vi "AXI-Stream-Tester-Top.vi"() -> ()   [LabVIEW 2017]
uses:
  AXI-Stream.States.ctl
  <vilib>/FPGAPlugInAG/PXIe-6592R/niLvFpga_Open_PXIe-6592R.vi
  <vilib>/rvi/interface/common/dynamic/niFpgaDynamicAddResources.vi
  AXI-Stream.Globals.vi
  <vilib>/Utility/error.llb/Error Cluster From Error Code.vi
  <vilib>/rvi/errors/niLvFpgaAdjustHostInterfaceError.vi
  <vilib>/FPGAPlugInAG/Dynamic/niLvFpga_Close_Dynamic.vi
  <vilib>/rvi/interface/nirviOpenFPGA/nirviOpenFPGA.xnode
  FPGA Bitfiles/03MicroBlazeAXIS_FPGATarget_Fpga-AXI-Stream_rt9YWQdBu5Q.lvbitx
  <vilib>/rvi/interface/nirviReadWriteControl/nirviReadWriteControl.xnode
  <vilib>/rvi/interface/nirviMethod/nirviMethod.xnode
  <vilib>/rvi/interface/nirviCloseFPGA/nirviCloseFPGA.xnode
  <vilib>/rvi/errors/niLvFpgaMergeErrorWithErrorCode.vi
  <vilib>/FPGAPlugInAG/Dynamic/niLvFpga_ReadFifo_Dynamic.vi
  <vilib>/rvi/interface/Simulation/niFpgaSimulationCallBeginRW.vi
  <vilib>/FPGAPlugInAG/Dynamic/niLvFpga_WriteFifo_Dynamic.vi
  NiFpgaLv.dll
panel:
  out "AXI_STR_RXD_tready_Count":u16
  out "TXD_tkeep_count 2":u32
  in  "AXI_STR_RXD_tuser":fxp<+,4,4>
  in  "AXI_STR_RXD_tkeep":fxp<+,4,4>
  out "AXI_STR_TXD_tuser":fxp<+,4,4>
  out "AXI_STR_TXD_tkeep":fxp<+,4,4>
  out "TXD_tkeep_count":u32
  out "TXD_tuser_count":u32
  in  "Clear?":bool
  out "GPIO #1 out":u32 format="%.0x"
  in  "GPIO #1 in":u32 format="%.0x"
  in  "Read from GPIO":bool
  in  "Write to GPIO":bool
  in  "Read from FIFO":bool
  out "error out":errorcluster
  out "Read Data":u32[](array[numeric]) format="%.0x"
  in  "DataToSend":u32[](array[numeric])=[240, 241, 242, 243, 244, 245] format="%.0x"
  in  "Send to FIFO":bool
  in  "Stop":bool
  in  "error in":errorcluster
  # "Send a packet of data, read the same data\necho'd back by MicroBlaze MCS"
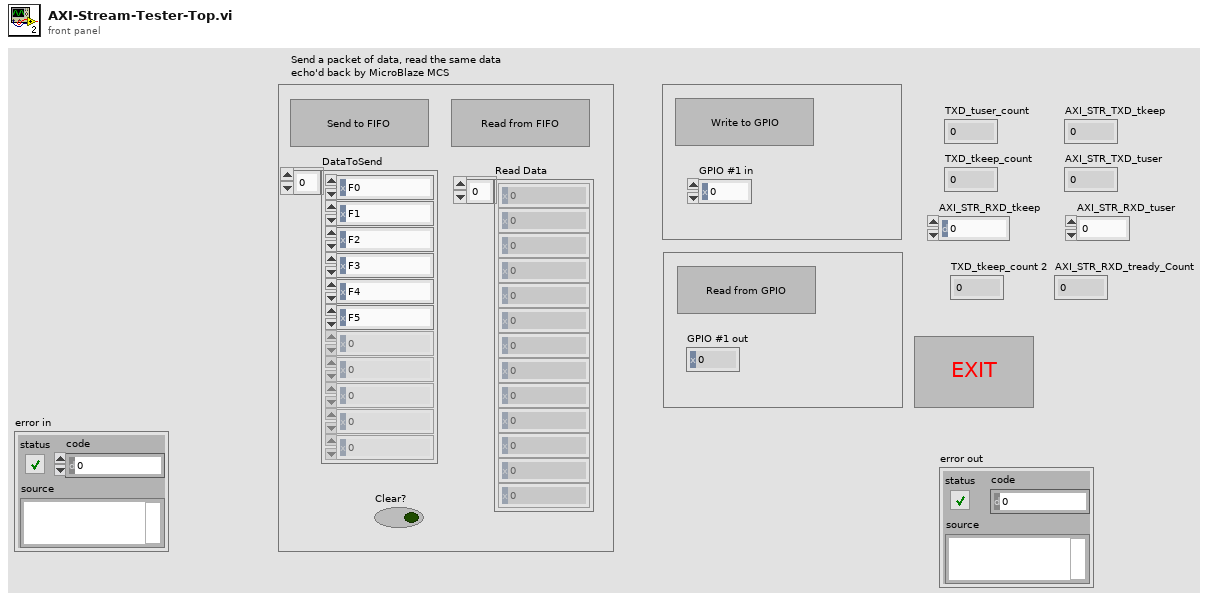
[diagram p1: front panel]
types:
  T1 = typedef "AXI-Stream.States.ctl" = enum16{"Open FPGA", "Send to FIFO", "Read from FIFO", "Write to GPIO", "Read GPIO", "Close FPGA"}
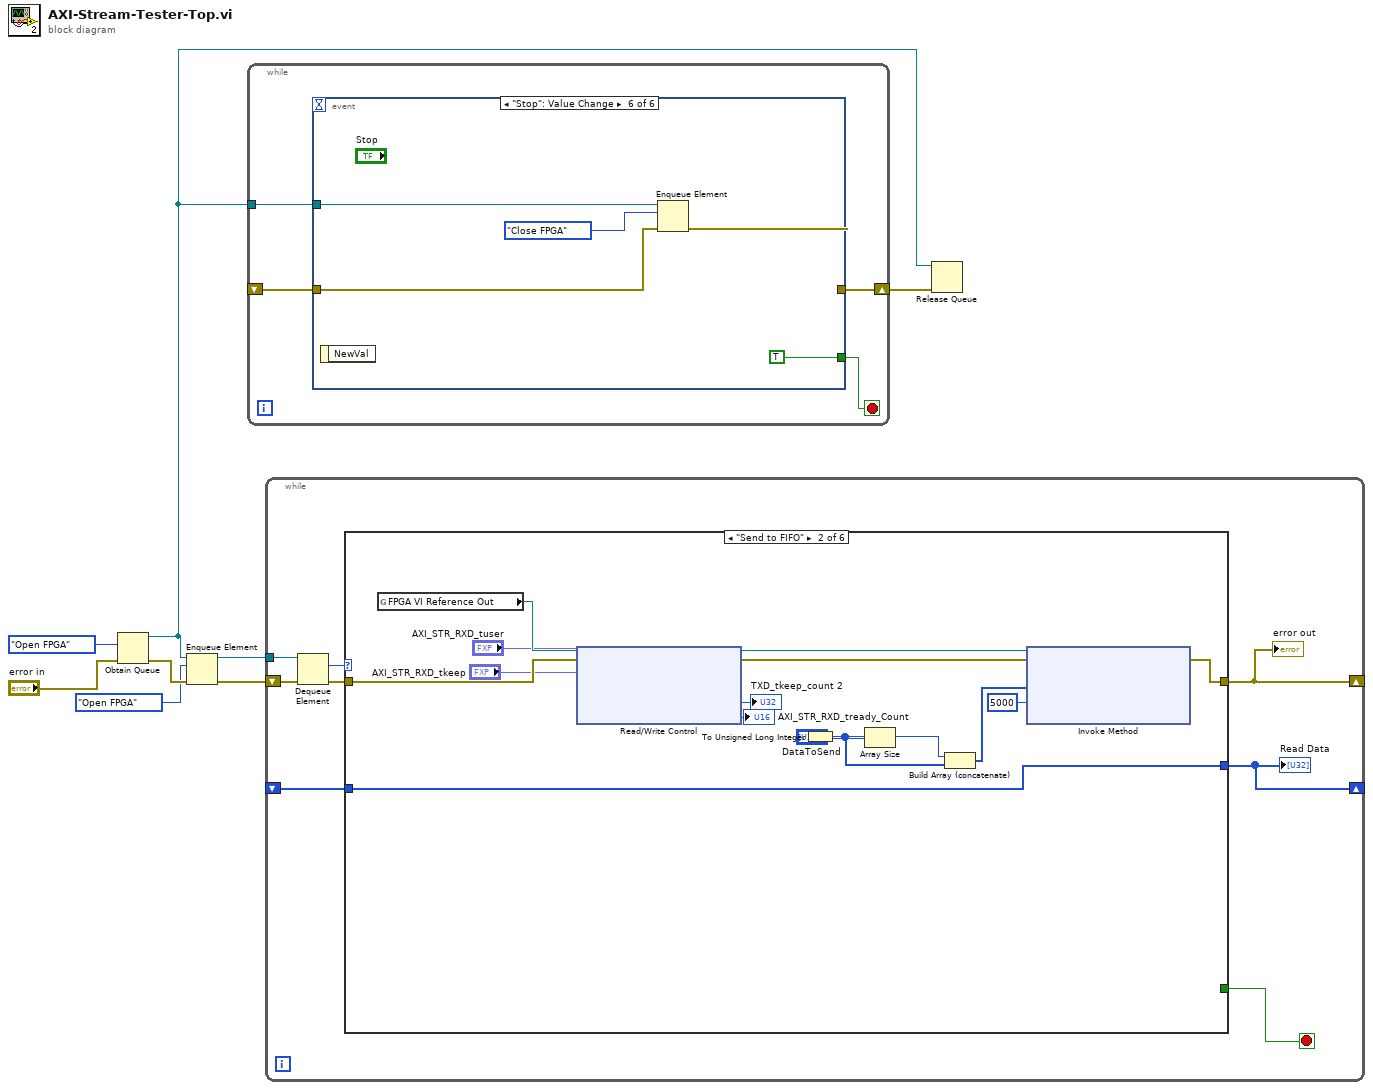
[diagram p0: block diagram]
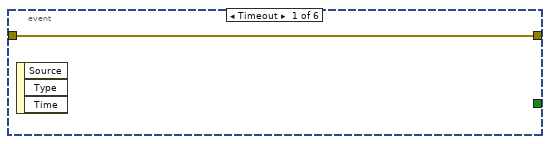
[diagram p2: hidden frame]
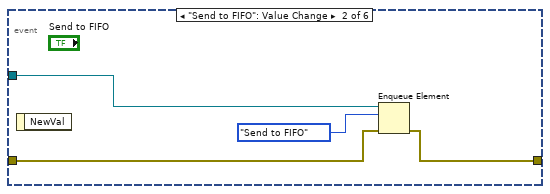
[diagram p3: hidden frame]
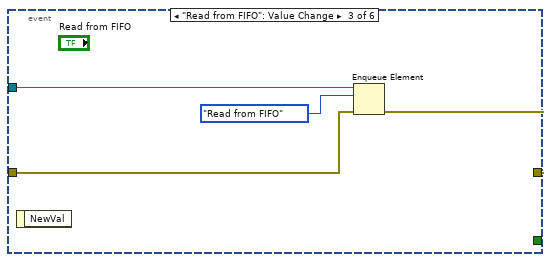
[diagram p4: hidden frame]
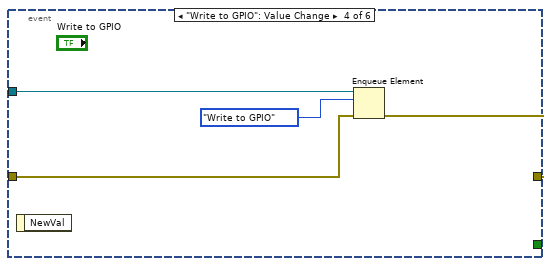
[diagram p5: hidden frame]
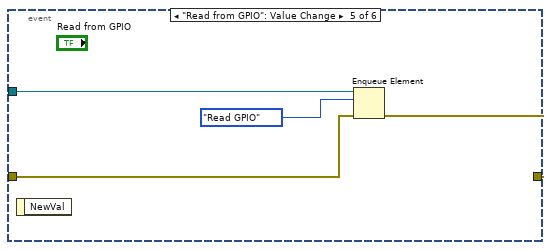
[diagram p6: hidden frame]
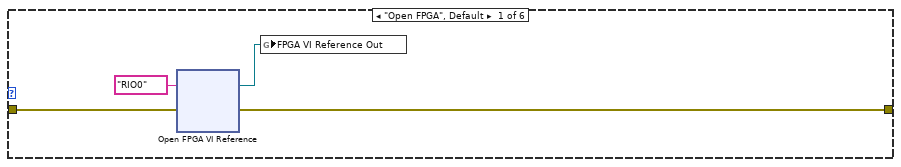
[diagram p7: hidden frame]
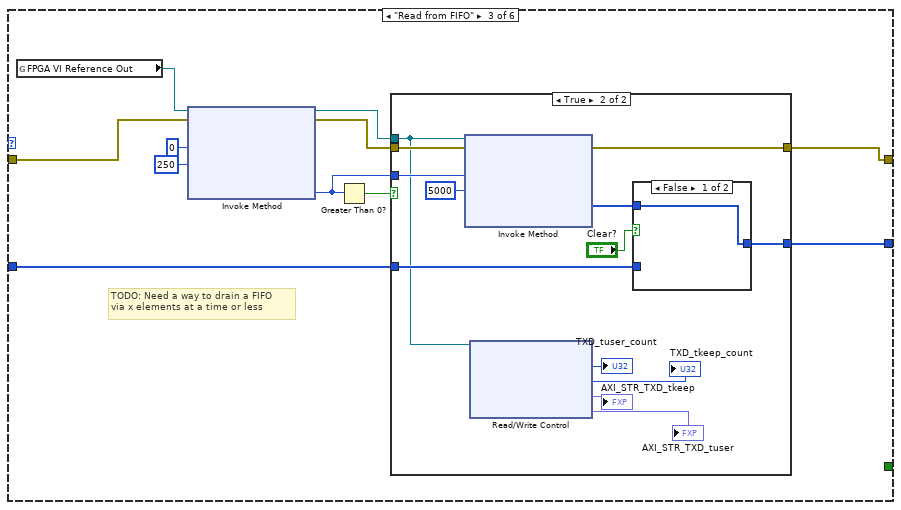
[diagram p8: hidden frame]
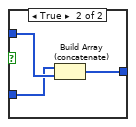
[diagram p10: hidden frame]
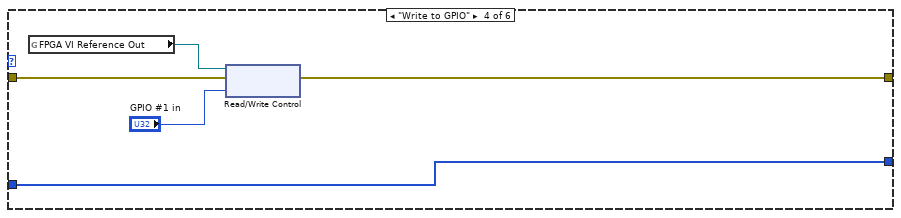
[diagram p11: hidden frame]
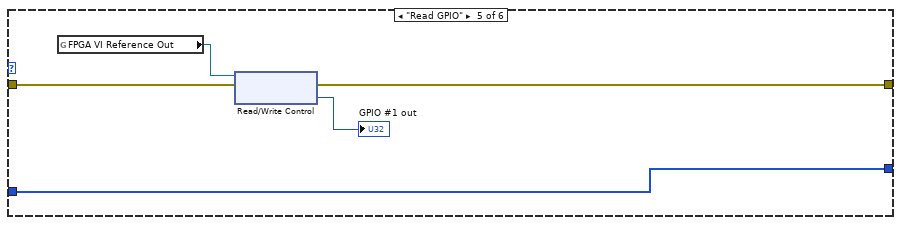
[diagram p12: hidden frame]
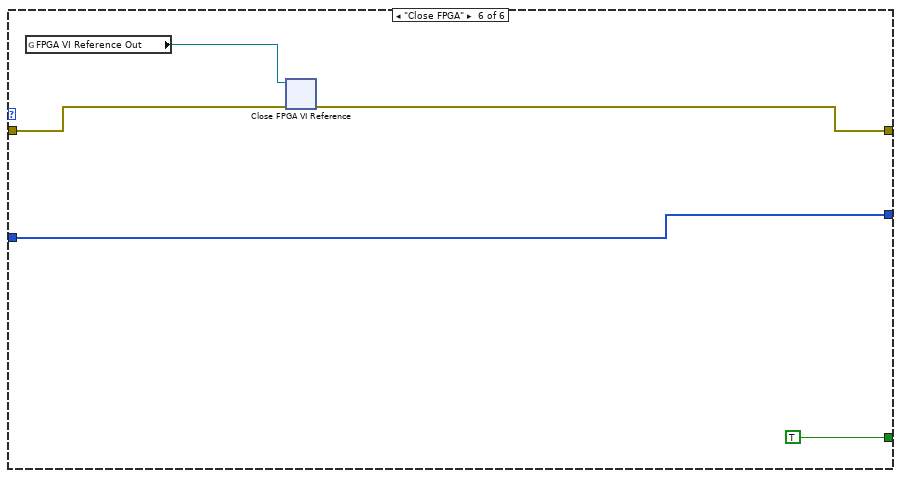
[diagram p13: hidden frame]
diagram:
  n1 = Obtain Queue(element data type=AXI-Stream.States."Open FPGA" ("Enum"), error in (no error)="error in") -> (queue out=w4:refnum<queue>, error out=w6:errorcluster)  [unwired: 3 in, 1 out]
  n2 = Enqueue Element(queue=w4, element=AXI-Stream.States."Open FPGA" ("Enum"), error in (no error)=w6) -> (queue out=w3:refnum<queue>, error out=w2:errorcluster)  [unwired: 1 in, 1 out]
  n3 = while {
    tunnel: w4 -> [w12]
    shift-right: [w11] -> w5
    shift-left: _ -> [w10]
    stop <- w9 stop-if-true
    n4 = event shown="[5] \"Stop\": Value Change" {
      selector: _ -> [_ _ _ _ _ _]
      dyn-events: _ -> [_ _ _ _ _ _]
      timeout: _ -> [_ _ _ _ _ _]
      tunnel: w12 -> [_ w17 w20 w24 w28 w33]
      tunnel: w10 -> [w13 w15 w19 w23 w27 w32]
      tunnel: [w13 w14 w18 w22 w26 w31] -> w11
      tunnel: [_ _ _ _ _ TRUE] -> w9
      event Timeout {
        n5 = event-data() -> ()  [unwired: 1 in, 3 out]
      }
      event "Send to FIFO": Value Change {
        n6 = event-data() -> ()  [unwired: 1 in, 1 out]
        n7 = Enqueue Element(queue=w17, element=AXI-Stream.States."Send to FIFO" ("Enum"), error in (no error)=w15) -> (error out=w14:errorcluster)  [unwired: 1 in, 2 out]
      }
      event "Read from FIFO": Value Change {
        n8 = event-data() -> ()  [unwired: 1 in, 1 out]
        n9 = Enqueue Element(queue=w20, element=AXI-Stream.States."Read from FIFO" ("Enum"), error in (no error)=w19) -> (error out=w18:errorcluster)  [unwired: 1 in, 2 out]
      }
      event "Write to GPIO": Value Change {
        n10 = event-data() -> ()  [unwired: 1 in, 1 out]
        n11 = Enqueue Element(queue=w24, element=AXI-Stream.States."Write to GPIO" ("Enum"), error in (no error)=w23) -> (error out=w22:errorcluster)  [unwired: 1 in, 2 out]
      }
      event "Read from GPIO": Value Change {
        n12 = event-data() -> ()  [unwired: 1 in, 1 out]
        n13 = Enqueue Element(queue=w28, element=AXI-Stream.States."Read GPIO" ("Enum"), error in (no error)=w27) -> (error out=w26:errorcluster)  [unwired: 1 in, 2 out]
      }
      event "Stop": Value Change {
        n14 = event-data() -> ()  [unwired: 1 in, 1 out]
        n15 = Enqueue Element(queue=w33, element=AXI-Stream.States."Close FPGA" ("Enum"), error in (no error)=w32) -> (error out=w31:errorcluster)  [unwired: 1 in, 2 out]
      }
    }
  }
  n16 = while {
    tunnel: w3 -> [w42]
    shift-right: [w38] -> _
    shift-left: w2 -> [w40]
    shift-right: [w37] -> _
    shift-left: _ -> [w36]
    stop <- w35 stop-if-true
    n17 = Dequeue Element(queue=w42, error in (no error)=w40) -> (element=w41:T1, error out=w39:errorcluster)  [unwired: 1 in, 2 out]
    n18 = case shown="\"Send to FIFO\"" w41 {
      tunnel: w39 -> [w46 w51 w69 w95 w100 w105]
      tunnel: [w44 w56 w65 w93 w98 w104] -> w38
      tunnel: [_ w55 w64 w92 w97 w103] -> w37
      tunnel: w36 -> [_ w55 w63 w92 w97 w103]
      tunnel: [_ _ _ _ _ TRUE] -> w35
      frame "Open FPGA", Default {
        n19 = xnode "Open FPGA VI Reference"("error in"=w46, "resource name"=tag "RIO0") -> ("FPGA VI Reference Out"=w43:refnum<k20>, "error out"=w44:errorcluster)
        n20 = global write "AXI-Stream.Globals.vi" "FPGA VI Reference Out"(w43) -> ()
      }
      frame "Send to FIFO" {
        n21 = global read "AXI-Stream.Globals.vi" "FPGA VI Reference Out"() -> (w54:refnum<k20>)
        n22 = xnode "Read/Write Control"("FPGA VI Reference In"=w54, "error in"=w51, "AXI_STR_RXD_tkeep"="AXI_STR_RXD_tkeep", "AXI_STR_RXD_tuser"="AXI_STR_RXD_tuser") -> ("FPGA VI Reference Out"=w53:refnum<k20>, "error out"=w52:errorcluster, "TXD_tkeep_count"=→"TXD_tkeep_count 2":u32, "AXI_STR_RXD_tready_Count"=→"AXI_STR_RXD_tready_Count":u16)
        n23 = Array Size(array="DataToSend") -> (size(s)=w59:i32)
        n24 = To Unsigned Long Integer(number=w59) -> (unsigned 32bit integer=w61:u32)
        n25 = Build Array (concatenate)(w61, "DataToSend") -> (w58:u32[])
        n26 = xnode "Invoke Method"("FPGA VI Reference In"=w53, "error in"=w52, "Data"=w58, "Timeout (ms)"=5000) -> ("error out"=w56:errorcluster)  [unwired: 2 out]
      }
      frame "Read from FIFO" {
        # "TODO: Need a way to drain a FIFO \nvia x elements at a time or less"
        n27 = global read "AXI-Stream.Globals.vi" "FPGA VI Reference Out"() -> (w72:refnum<k20>)
        n28 = xnode "Invoke Method"("FPGA VI Reference In"=w72, "error in"=w69, "Number of Elements"=u32 0, "Timeout (ms)"=250) -> ("FPGA VI Reference Out"=w62:refnum<k20>, "error out"=w66:errorcluster, "Elements Remaining"=w67:u32)  [unwired: 1 out]
        n29 = Greater Than 0?(x=w67) -> (x > 0?=w68:bool)
        n30 = case shown="True" w68 {
          tunnel: w67 -> [_ w87]
          tunnel: w66 -> [w74 w85]
          tunnel: [w74 w84] -> w65
          tunnel: [w73 w83] -> w64
          tunnel: w63 -> [w73 w81]
          tunnel: w62 -> [_ w79]
          frame False {
          }
          frame True {
            n31 = xnode "Invoke Method"("FPGA VI Reference In"=w79, "error in"=w85, "Number of Elements"=w87, "Timeout (ms)"=5000) -> ("error out"=w84:errorcluster, "Data"=w82:u32[])  [unwired: 2 out]
            n32 = xnode "Read/Write Control"("FPGA VI Reference In"=w79) -> ("TXD_tuser_count"=→"TXD_tuser_count":u32, "TXD_tkeep_count"=→"TXD_tkeep_count":u32, "AXI_STR_TXD_tkeep"=→"AXI_STR_TXD_tkeep":fxp<+,4,4>, "AXI_STR_TXD_tuser"=→"AXI_STR_TXD_tuser":fxp<+,4,4>)  [unwired: 1 in, 2 out]
            n33 = case shown="False" "Clear?" {
              tunnel: [w88 w91] -> w83
              tunnel: w82 -> [w88 w90]
              tunnel: w81 -> [_ w89]
              frame False {
              }
              frame True {
                n34 = Build Array (concatenate)(w89, w90) -> (w91:u32[])
              }
            }
          }
        }
      }
      frame "Write to GPIO" {
        n35 = global read "AXI-Stream.Globals.vi" "FPGA VI Reference Out"() -> (w96:refnum<k20>)
        n36 = xnode "Read/Write Control"("FPGA VI Reference In"=w96, "error in"=w95, "GPIO #1 in"="GPIO #1 in") -> ("error out"=w93:errorcluster)  [unwired: 1 out]
      }
      frame "Read GPIO" {
        n37 = global read "AXI-Stream.Globals.vi" "FPGA VI Reference Out"() -> (w101:refnum<k20>)
        n38 = xnode "Read/Write Control"("FPGA VI Reference In"=w101, "error in"=w100) -> ("error out"=w98:errorcluster, "GPIO #1 out"=→"GPIO #1 out":u32)  [unwired: 1 out]
      }
      frame "Close FPGA" {
        n39 = global read "AXI-Stream.Globals.vi" "FPGA VI Reference Out"() -> (w106:refnum<k20>)
        n40 = xnode "Close FPGA VI Reference"("FPGA VI Reference In"=w106, "error in"=w105) -> ("error out"=w104:errorcluster)
      }
    }
    "error out" <- w38
    "Read Data" <- w37
  }
  n41 = Release Queue(queue=w4, error in (no error)=w5) -> ()  [unwired: 1 in, 3 out]
